vi "sortTetRecChannels.vi"(8 "error in (no error)":errorcluster, 11 "shared variable refnum in":refnum<k21>="ni.var.psp://at-s1no1/AcquisitionVariables/ChannelNames") -> (0 "error out":errorcluster, 1 "sortedTetNum":i32[](array[numeric]), 2 "sortedTetChanNum":i32[](array[numeric]), 3 "sortedChanIdx":i32[](array[numeric]), 4 "unsortedChanNum":i32[](array[numeric]), 5 "reorderedChanNums":i32[](array[numeric]), 6 "unsortedTetNums":i32[](array[numeric]))   [LabVIEW 2010]
uses:
  <vilib>/regexp/Match Regular Expression.xnode
  <vilib>/imath/engines/lvmath2/RunTimeEngine/ErrorHandling/NIMS_Finalize Error.vi
  <vilib>/imath/engines/lvmath2/RunTimeEngine/BuiltInFunctions/sort/NIMS_[2o]_sort(RRowV,I32,Str).vi
  <instcachedir>/0/NIMS_[2o]_sort(RRowV,I32,Str)_1834406CABAC430BB40FEC772A4FC192.lvgen/NIMS_[2o]_sort(RRowV,I32,Str)_1834406CABAC430BB40FEC772A4FC192_001.vi
  <vilib>/imathl/engines/lvmath/Functions/Error Handling/Create Error.vi
  <vilib>/imath/engines/lvmath2/RunTimeEngine/NodeEndStatement/NIMS_NodeEndStatement_Output.vi
  <instcachedir>/0/NIMS_NodeEndStatement_Output_53EC0D466D134D7ABD903AC30B43404B.lvgen/NIMS_NodeEndStatement_Output_53EC0D466D134D7ABD903AC30B43404B_005.vi
  <instcachedir>/0/NIMS_NodeEndStatement_Output_53EC0D466D134D7ABD903AC30B43404B.lvgen/NIMS_NodeEndStatement_Output_53EC0D466D134D7ABD903AC30B43404B_004.vi
  <vilib>/imath/engines/lvmath2/RunTimeEngine/VariableToken/Read/NIMS_Get Elements - RV(_) - Check.vi
  <instcachedir>/0/NIMS_Get Elements - RV(_) - Check_1F6F8656162345078B1D4DC9877DFAE9.lvgen/NIMS_Get Elements - RV(_) - Check_1F6F8656162345078B1D4DC9877DFAE9_003.vi
  <vilib>/imath/engines/lvmath2/RunTimeEngine/BuiltInFunctions/length/NIMS_length(GV).vi
  <instcachedir>/0/NIMS_length(GV)_08A3D13377FD4E4B96F5795FBF3698FA.lvgen/NIMS_length(GV)_08A3D13377FD4E4B96F5795FBF3698FA_002.vi
  <vilib>/imath/engines/lvmath2/RunTimeEngine/ReplaceToken/NIMS_Replace - Check Linear.vi
  <instcachedir>/0/NIMS_Replace - Check Linear_662D5651E4E34E0584DA82A256193A4C.lvgen/NIMS_Replace - Check Linear_662D5651E4E34E0584DA82A256193A4C_007.vi
  <vilib>/imath/engines/lvmath2/RunTimeEngine/RangeToken/NIMS_Range.vi
  <instcachedir>/0/NIMS_Range_1C63927E4E474DADACDA97C3F2261A11.lvgen/NIMS_Range_1C63927E4E474DADACDA97C3F2261A11_000.vi
  <vilib>/imath/engines/lvmath2/RunTimeEngine/ReplaceToken/NIMS_Replace - Size Check _(_)=VorM.vi
  <instcachedir>/0/NIMS_Replace - Size Check _(_)=VorM_4228B35EE910471DB74F3866D9D09B95.lvgen/NIMS_Replace - Size Check _(_)=VorM_4228B35EE910471DB74F3866D9D09B95_007.vi
  <vilib>/imath/engines/lvmath2/RunTimeEngine/ReplaceToken/NIMS_Replace - Assignment Check _(_)=VorM.vi
  <instcachedir>/0/NIMS_Replace - Assignment Check _(_)=VorM_C130F3B8B64B4DD7B9359A2D3A035D18.lvgen/NIMS_Replace - Assignment Check _(_)=VorM_C130F3B8B64B4DD7B9359A2D3A035D18_007.vi
  <vilib>/imath/engines/lvmath2/RunTimeEngine/ErrorHandling/NIMS_Create Error From Enums.vi
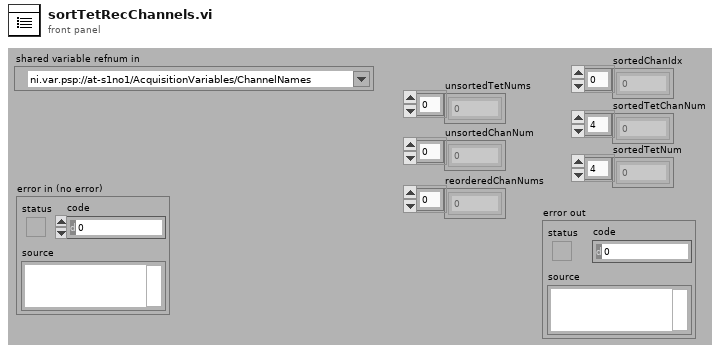
[diagram p1: front panel]
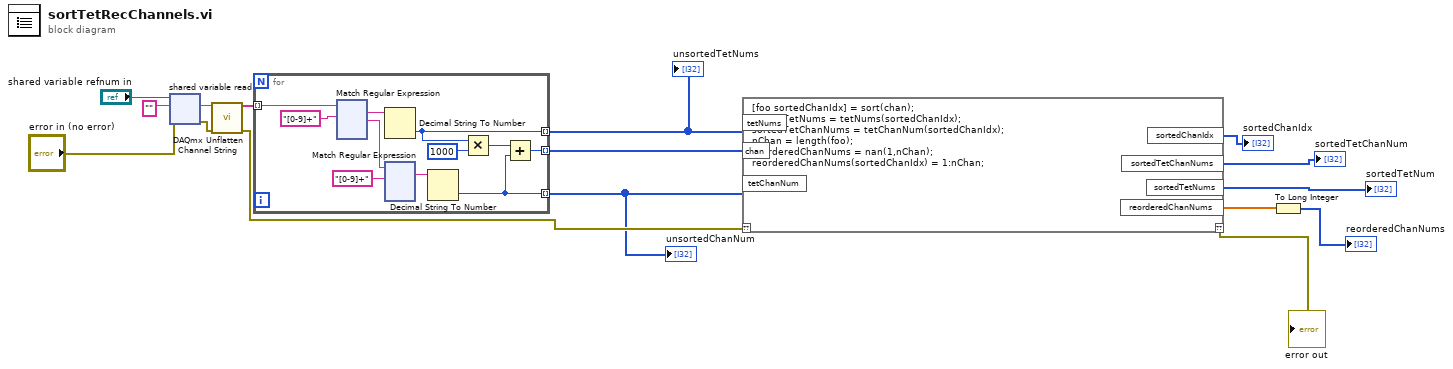
[diagram p0: block diagram]
diagram:
  n1 = shared-variable-read("shared variable refnum in", "error in (no error)", "") -> (w10:errorcluster, w14:string)  [unwired: 2 out]
  n2 = call <vilib>:"DAQmx Unflatten Channel String.vi"("names in"=w14, "error in"=w10) -> ("names out"=w13:string[], "error out"=w9:errorcluster)  [unwired: 12 in]
  n3 = for {
    tunnel: w13 -> [w26] mode=indexing
    tunnel: [w19] -> w6 mode=indexing
    tunnel: [w18] -> w12 mode=indexing
    tunnel: [w17] -> w7 mode=indexing
    n4 = xnode "Match Regular Expression"("input string"=w26, "regular expression"="[0-9]+") -> ("whole match"=w23:string, "after match"=w24:string)  [unwired: 4 in, 3 out]
    n5 = Decimal String To Number(string=w23) -> (number=w18:i32)  [unwired: 2 in, 1 out]
    n6 = xnode "Match Regular Expression"("input string"=w24, "regular expression"="[0-9]+") -> ("whole match"=w22:string)  [unwired: 4 in, 4 out]
    n7 = Decimal String To Number(string=w22) -> (number=w17:i32)  [unwired: 2 in, 1 out]
    n8 = Multiply(x=w18, y=1000) -> (x*y=w20:i32)
    n9 = Add(x=w20, y=w17) -> (x+y=w19:i32)
  }
  "unsortedTetNums" <- w12
  "unsortedChanNum" <- w7
  n10 = mathscript code="[foo sortedChanIdx] = sort(chan);\nsortedTetNums = tetNums(sortedChanIdx);\nsortedTetChanNums = tetChanNum(sortedChanIdx);\nnChan = length(foo);\nreorderedChanNums = nan(1,nChan);\nreorderedChanNums(sortedChanIdx) = 1:nChan;"("??"=w9, "chan"=w6, "tetNums"=w12, "tetChanNum"=w7) -> ("??"=→"error out":errorcluster, "sortedTetChanNums"=→"sortedTetChanNum":i32[], "sortedTetNums"=→"sortedTetNum":i32[], "sortedChanIdx"=→"sortedChanIdx":i32[], "reorderedChanNums"=w2:dbl[])
  n11 = To Long Integer(number=w2) -> (32bit integer=→"reorderedChanNums":i32[])
